vi "Read condtional.vi"(9 "ForLoop in":refnum<class "WhileLoop.lvclass">) -> (3 "ForLoop out":refnum<class "WhileLoop.lvclass">, 4 "condtional":bool)   [LabVIEW 2014]
uses:
  WhileLoop.lvclass
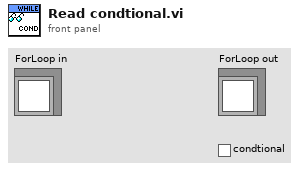
[diagram p1: front panel]
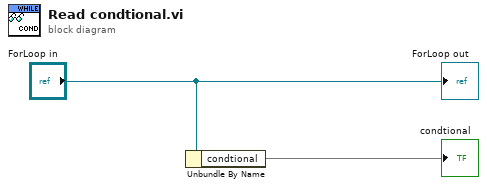
[diagram p0: block diagram]
diagram:
  n1 = Unbundle By Name("ForLoop in") -> ("condtional"=→"condtional")
  "ForLoop out" <- "ForLoop in"
